vi "minivia.vi"(7 "Minify Locals?":bool, 9 "Remove JavaScriptInvoke":bool=TRUE, 10 "Remove Whitespace":bool, 11 "VIA":string="// Autogenerated Vireo assembly file\n// Generated on 07/31/2021 00:31:29\n//---------------------------------------------------\n//VI Definition: ::Web Server::Interactive::HelloBlink::HelloBlink.gviweb\ndefine (HelloBlink%3A%3AHelloBlink%2Egviweb dv(.VirtualInstrument (\n    Locals: c(   // Data Space\n        e(dv(.String 'HelloBlink::HelloBlink.gviweb')local0)\n        ce(dv(.Boolean true)c1)\n        ce(dv(.UInt32 25)c2)\n        e(.Int32 local3)\n        ce(dv(.Boolean false)c4)\n        ce(dv(.UInt32 1000)c5)\n        ce(dv(.String 'Hello LabWorld %d')c6)\n        e(.String local7)\n        e(.UInt32 local8)\n        e(.UInt32 local9)\n        e(.UInt32 local10)\n        e(.Int32 local11)\n        e(.Boolean local12)\n        e(.Boolean local13)\n        e(.Boolean local14)\n        ce(dv(.Boolean false)c15)\n        ce(dv(.UInt32 500)c16)\n        e(.UInt32 local17)\n        e(.UInt32 local18)\n        ce(dv(.Int32 0)c19)\n        e(.Int32 local20)\n        ce(dv(.Int32 2147483647)c21)\n        ce(dv(.Int32 0)c22)\n        e(.UInt32 local23)\n        ce(dv(.Int32 2147483647)c24)\n    )\n        clump(1\n        Trigger(1)\n        Trigger(2)\n        Wait(1)\n        Wait(2)\n/* Clump Ended. */    )\n    clump(1\n        PicoGLib%3A%3AGPIO%3A%3AInit%2Egvi(c2 local9)\n        PicoGLib%3A%3AGPIO%3A%3ASetOutput%2Egvi(local9 c1 local10)\n        Copy(c1 local13)\n        Copy(c22 local11)\n        Copy(local10 local23)\n    Perch(0)\n        Copy(local13 local12)\n        Not(local12 local14 )\n        Trigger(5)\n        Trigger(6)\n        Wait(5)\n        Wait(6)\n        Copy(local14 local13)\n        BranchIfTrue(1 c15)\n        BranchIfEQ(0 local11 c24)\n        Increment(local11 local11 )\n        Branch(0)\n    Perch(1)\n        // Code End\n/* Clump Ended. */    )\n    clump(1\n        Copy(c19 local3)\n    Perch(0)\n        StringFormatValue(local7 c6 local3 )\n        Trigger(3)\n        Trigger(4)\n        Wait(3)\n        Wait(4)\n        Copy(local3 local20)\n        BranchIfTrue(1 c4)\n        BranchIfEQ(0 local3 c21)\n        Increment(local3 local3 )\n        Branch(0)\n    Perch(1)\n        // Code End\n/* Clump Ended. */    )\n    clump(1\n        PicoGLib%3A%3ACore%3A%3APrintln%2Egvi(local7)\n        // Code End\n/* Clump Ended. */    )\n    clump(1\n        WaitMilliseconds(c5 * )\n        // Code End\n/* Clump Ended. */    )\n    clump(1\n        PicoGLib%3A%3AGPIO%3A%3AWrite%2Egvi(local10 local12 *)\n        // Code End\n/* Clump Ended. */    )\n    clump(1\n        WaitMilliseconds(c16 * )\n        // Code End\n/* Clump Ended. */    )\n)))\n// Autogenerated Vireo assembly file\n// Generated on 07/31/2021 00:29:56\n//---------------------------------------------------\n//VI Definition: ::Web Server::Interactive::PicoGLib::GPIO::Write.gvi\ndefine (PicoGLib%3A%3AGPIO%3A%3AWrite%2Egvi dv(.VirtualInstrument (\n    Params: c(  //param block\n        i(dv(.UInt32 0)dataItem_PinIn)\n        i(dv(.Boolean false)dataItem_Value)\n        o(dv(.UInt32 0)dataItem_PinPinIn)\n    )\n    Locals: c(   // Data Space\n        e(dv(.String 'PicoGLib::GPIO::Write.gvi')local3)\n        e(.Boolean local4)\n        e(.UInt32 local5)\n        e(.UInt32 local6)\n    )\n        clump(1\n        Copy(dataItem_PinIn local5)\n        Copy(local5 dataItem_PinPinIn)\n/* Clump Ended. */    )\n)))\n// Autogenerated Vireo assembly file\n// Generated on 07/31/2021 00:29:56\n//---------------------------------------------------\n//VI Definition: ::Web Server::Interactive::PicoGLib::GPIO::SetOutput.gvi\ndefine (PicoGLib%3A%3AGPIO%3A%3ASetOutput%2Egvi dv(.VirtualInstrument (\n    Params: c(  //param block\n        i(dv(.UInt32 0)dataItem_PinIn)\n        i(dv(.Boolean false)dataItem_Output)\n        o(dv(.UInt32 0)dataItem_PinPinIn)\n    )\n    Locals: c(   // Data Space\n        e(dv(.String 'PicoGLib::GPIO::SetOutput.gvi')local3)\n        e(.Boolean local4)\n        e(.UInt32 local5)\n        e(.UInt32 local6)\n    )\n        clump(1\n        Copy(dataItem_PinIn local5)\n        Copy(local5 dataItem_PinPinIn)\n/* Clump Ended. */    )\n)))\n// Autogenerated Vireo assembly file\n// Generated on 07/31/2021 00:29:56\n//---------------------------------------------------\n//VI Definition: ::Web Server::Interactive::PicoGLib::GPIO::Init.gvi\ndefine (PicoGLib%3A%3AGPIO%3A%3AInit%2Egvi dv(.VirtualInstrument (\n    Params: c(  //param block\n        i(dv(.UInt32 0)dataItem_PinIn)\n        o(dv(.UInt32 0)dataItem_PinPinIn)\n    )\n    Locals: c(   // Data Space\n        e(dv(.String 'PicoGLib::GPIO::Init.gvi')local2)\n        e(.UInt32 local3)\n        e(.UInt32 local4)\n    )\n        clump(1\n        Copy(dataItem_PinIn local3)\n        Copy(local3 dataItem_PinPinIn)\n/* Clump Ended. */    )\n)))\n// Autogenerated Vireo assembly file\n// Generated on 07/31/2021 00:31:10\n//---------------------------------------------------\n//VI Definition: ::Web Server::Interactive::PicoGLib::Core::Println.gvi\ndefine (PicoGLib%3A%3ACore%3A%3APrintln%2Egvi dv(.VirtualInstrument (\n    Params: c(  //param block\n        i(dv(.String '')dataItem_String)\n    )\n    Locals: c(   // Data Space\n        e(dv(.String 'PicoGLib::Core::Println.gvi')local1)\n        e(.String local2)\n    )\n        clump(1\n/* Clump Ended. */    )\n)))\nenqueue (HelloBlink%3A%3AHelloBlink%2Egviweb)\n//Finished!! :D\n") -> (3 "Minified":string)   [LabVIEW 2020]
uses:
  <vilib>/regexp/Match Regular Expression.xnode
panel:
  out "% saved":dbl
  out "length":i32
  in  "Remove Enqueue?":bool
  in  "Rename Top-Level (Blank = as-is)":string="main"
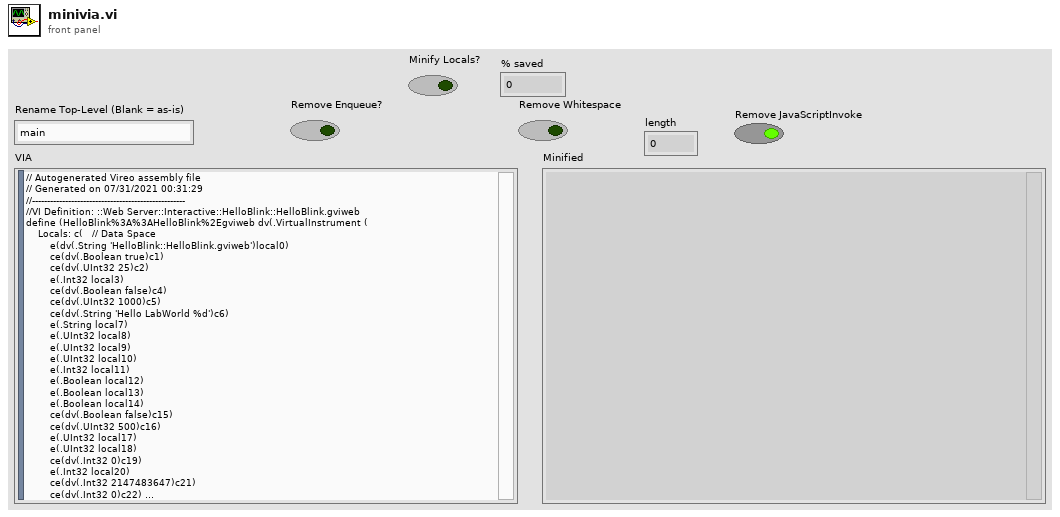
[diagram p1: front panel]
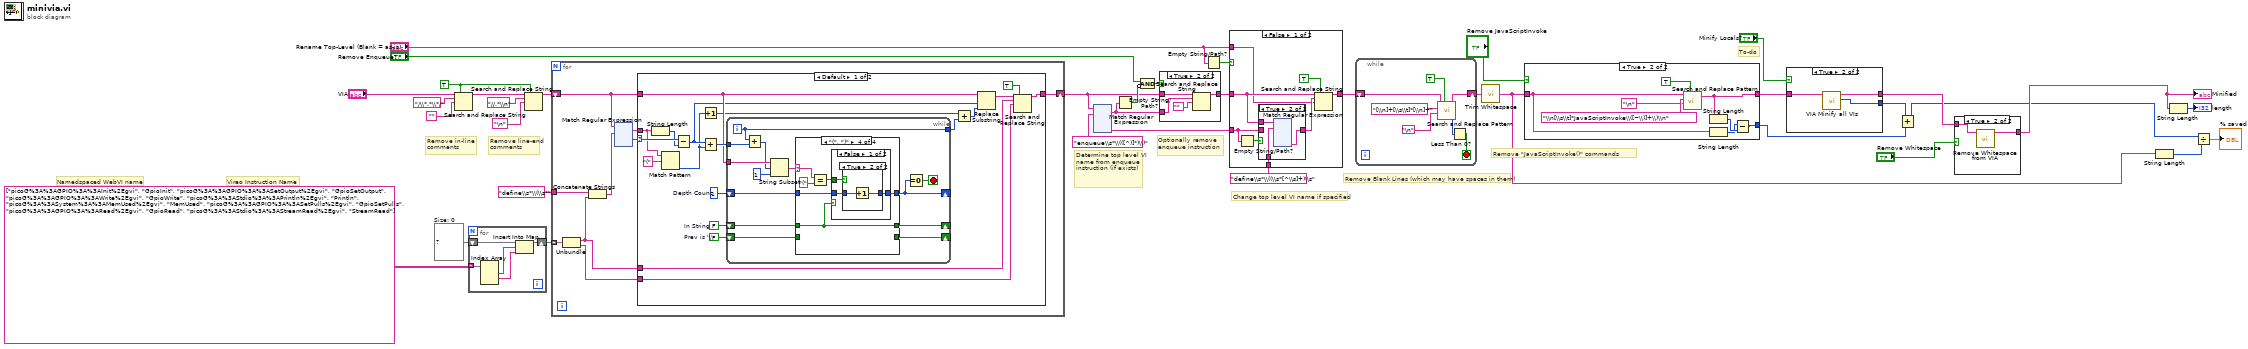
[diagram p0: block diagram]
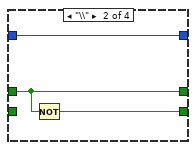
[diagram p6: hidden frame]
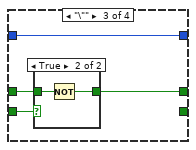
[diagram p7: hidden frame]
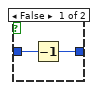
[diagram p9: hidden frame]
diagram:
  w17 = map{string, string} {}  # Size: 0
  w34 = TRUE ("replace all? (F)")
  # "Remove \"JavaScriptInvoke()\" commands"
  # "Remove Blank Lines (which may have spaces in them)"
  # "Vireo Instruction Name"
  # "Namedspaced WebVI name"
  # "To-do"
  # "Change top level VI name if specified"
  # "Optionally remove enqueue instruction"
  # "Determine top level VI name from enqueue instruction (if exists)"
  # "Remove line-end comments"
  # "Remove in-line comments"
  n1 = Search and Replace String(replace all?=w34, input string="VIA", search string="/\\*.*\\*/", replace string="") -> (result string=w36:string)  [unwired: 4 in, 3 out]
  n2 = for {
    tunnel: string[][] [["picoG%3A%3AGPIO%3A%3AInit%2Egvi", "GpioInit"], ["picoG%3A%3AGPIO%3A%3ASetOutput%2Egvi", "GpioSetOutput"], ["picoG%3A%3AGPIO%3A%3AWrite%2Egvi", "GpioWrite"], ["picoG%3A%3AStdio%3A%3APrintln%2Egvi", "Println"], ["picoG%3A%3ASystem%3A%3AMemUsed%2Egvi", "MemUsed"], ["picoG%3A%3AGPIO%3A%3ASetPulls%2Egvi", "GpioSetPulls"], ["picoG%3A%3AGPIO%3A%3ARead%2Egvi", "GpioRead"], ["picoG%3A%3AStdio%3A%3AStreamRead%2Egvi", "StreamRead"]] -> [w42] mode=indexing
    shift-right: [w40] -> w20
    shift-left: w17 -> [w43]
    n3 = Index Array(array=w42) -> (element #1=w41:string, element #2=w39:string)  [unwired: 3 in, 1 out]
    n4 = Insert Into Map(map in=w43, key=w41, value=w39) -> (map out=w40:map{string, string})  [unwired: 2 out]
  }
  n5 = Search and Replace String(replace all?=w34, input string=w36, search string="//.*\\n", replace string="\n") -> (result string=w21:string)  [unwired: 4 in, 3 out]
  n6 = for {
    shift-right: [w47] -> w18
    shift-left: w21 -> [w48]
    tunnel: w20 -> [w52] mode=indexing
    tunnel: "define\\s*\\(\\s*" -> [w51]
    n7 = Unbundle(w52) -> (w44:string, w45:string)
    n8 = Concatenate Strings(w51, w44) -> (w50:string)
    n9 = xnode "Match Regular Expression"("input string"=w48, "regular expression"=w50) -> ("whole match"=w46:string, "offset past match"=w49:i32)  [unwired: 4 in, 3 out]
    n10 = case shown="Default" w49 {
      selector: w49 -> [w71 _]
      tunnel: w48 -> [w64 w111]
      tunnel: [w54 w111] -> w47
      tunnel: w46 -> [w69 _]
      tunnel: w45 -> [w58 _]
      tunnel: w44 -> [w56 _]
      frame Default {
        w53 = FALSE  # Prev is '\'
        w65 = FALSE  # In String
        w67 = 1  # Depth Count
        n11 = String Length(string=w69) -> (length=w70:i32)
        n12 = Match Pattern(string=w69, regular expression="(") -> (offset past match=w61:i32)  [unwired: 1 in, 3 out]
        n13 = Subtract(x=w71, y=w70) -> (x-y=w63:i32)
        n14 = Increment(x=w61) -> (x+1=w59:i32)
        n15 = Add(x=w63, y=w61) -> (x+y=w66:i32)
        n16 = while {
          shift-right: [w76] -> _
          shift-left: w67 -> [w80]
          tunnel: w66 -> [w84]
          tunnel: w64 -> [w83]
          shift-right: [w73] -> _
          shift-left: w65 -> [w78]
          shift-right: [w74] -> _
          shift-left: w53 -> [w77]
          tunnel: [w72] -> w62
          i -> [w72]
          stop <- w75 stop-if-true
          n17 = Add(x=w72, y=w84) -> (x+y=w82:i32)
          n18 = String Subset(string=w83, offset (0)=w82, length (rest)=1 ("length (rest)")) -> (substring=w79:string)
          n19 = case shown="\"(\", \")\"" w79 {
            selector: w79 -> [_ _ _ w100]
            tunnel: w80 -> [w86 w88 w90 w102]
            tunnel: [w86 w88 w90 w101] -> w76
            tunnel: w78 -> [w85 w87 w92 w98]
            tunnel: w77 -> [_ _ w93 _]
            tunnel: [_ w89 _ _] -> w74
            tunnel: [w85 w87 w91 w98] -> w73
            frame Default {
            }
            frame "\\" {
              n20 = Not(x=w87) -> (.not. x?=w89:bool)
            }
            frame "\"" {
              n21 = case shown="True" w93 {
                tunnel: w92 -> [w94 w96]
                tunnel: [w94 w95] -> w91
                frame False {
                }
                frame True {
                  n22 = Not(x=w96) -> (.not. x?=w95:bool)
                }
              }
            }
            frame "(", ")" {
              n23 = Equal?(x=w100, y="(") -> (x = y?=w97:bool)
              n24 = case shown="False" w98 {
                tunnel: w102 -> [w105 w110]
                tunnel: [w104 w110] -> w101
                tunnel: w97 -> [w103 _]
                frame False {
                  n25 = case shown="True" w103 {
                    tunnel: w105 -> [w107 w109]
                    tunnel: [w106 w108] -> w104
                    frame False {
                      n26 = Decrement(x=w107) -> (x-1=w106:i32)
                    }
                    frame True {
                      n27 = Increment(x=w109) -> (x+1=w108:i32)
                    }
                  }
                }
                frame True {
                }
              }
            }
          }
          n28 = Equal To 0?(x=w76) -> (x = 0?=w75:bool)
        }
        n29 = Add(x=w59, y=w62) -> (x+y=w60:i32)
        n30 = Replace Substring(2:w60, 3:w63, 5:w64) -> (1:w57:string)  [unwired: 1 in, 1 out]
        n31 = Search and Replace String(replace all?=TRUE ("replace all? (F)"), input string=w57, search string=w56, replace string=w58) -> (result string=w54:string)  [unwired: 4 in, 3 out]
      }
      frame -1 {
        # "Built-in not used"
      }
    }
  }
  n32 = xnode "Match Regular Expression"("input string"=w18, "regular expression"="enqueue\\s*\\(([^)]*)\\)") -> ("whole match"=w30:string, "submatch 1"=w27:string)  [unwired: 4 in, 4 out]
  n33 = Empty String/Path?(string/path=w30) -> (empty?=w29:bool)
  n34 = Compound Arithmetic op=AND("Remove Enqueue?", invert w29) -> (w28:bool)
  n35 = case shown="True" w28 {
    tunnel: w18 -> [w226 w230]
    tunnel: w30 -> [_ w228]
    tunnel: [w226 w229] -> w26
    frame False {
    }
    frame True {
      n36 = Search and Replace String(input string=w230, search string=w228, replace string="") -> (result string=w229:string)  [unwired: 5 in, 3 out]
    }
  }
  n37 = Empty String/Path?(string/path="Rename Top-Level (Blank = as-is)") -> (empty?=w25:bool)
  n38 = case shown="False" w25 {
    tunnel: w27 -> [w236 _]
    tunnel: w26 -> [w235 w359]
    tunnel: [w234 w359] -> w15
    tunnel: "define\\s*\\((\\s*[^\\s]+)\\s" ("regular expression") -> [w237 _]
    tunnel: "Rename Top-Level (Blank = as-is)" -> [w231 _]
    frame False {
      n39 = Empty String/Path?(string/path=w236) -> (empty?=w238:bool)
      n40 = case shown="True" w238 {
        tunnel: w235 -> [_ w242]
        tunnel: w237 -> [_ w241]
        tunnel: w236 -> [w239 _]
        tunnel: [w239 w240] -> w232
        frame False {
        }
        frame True {
          n41 = xnode "Match Regular Expression"("input string"=w242, "regular expression"=w241) -> ("submatch 1"=w240:string)  [unwired: 4 in, 5 out]
        }
      }
      n42 = Search and Replace String(replace all?=TRUE ("replace all? (F)"), input string=w235, search string=w232, replace string=w231) -> (result string=w234:string)  [unwired: 4 in, 3 out]
    }
    frame True {
    }
  }
  n43 = while {
    shift-right: [w363] -> w6
    shift-left: w15 -> [w364]
    stop <- w360 stop-if-true
    n44 = call <vilib>:"Search and Replace Pattern.vi"("string"=w364, "regular expression (\"\")"="[\\n]+[\\s\\t]*[\\n]+" ("regular expression (\"\")"), "replace string (\"\")"="\n", "replace all? (F)"=TRUE) -> ("result string"=w363:string, "offset past match"=w361:i32)  [unwired: 1 in]
    n45 = Less Than 0?(x=w361) -> (x < 0?=w360:bool)
  }
  n46 = call <vilib>:"Trim Whitespace.vi"("string"=w6) -> ("trimmed string"=w4:string)  [unwired: 1 in]
  n47 = case shown="True" "Remove JavaScriptInvoke" {
    tunnel: w4 -> [w367 w371]
    tunnel: [w367 w372] -> w5
    tunnel: [_ w368] -> w3
    frame False {
    }
    frame True {
      n48 = call <vilib>:"Search and Replace Pattern.vi"("string"=w371, "regular expression (\"\")"="\\n[\\s\\t]*JavaScriptInvoke\\([~\\)]+\\)\\n" ("regular expression (\"\")"), "replace string (\"\")"="\n" ("replace string (\"\")"), "replace all? (F)"=TRUE) -> ("result string"=w372:string)  [unwired: 1 in, 1 out]
      n49 = String Length(string=w372) -> (length=w370:i32)
      n50 = String Length(string=w371) -> (length=w369:i32)
      n51 = Subtract(x=w369, y=w370) -> (x-y=w368:i32)
    }
  }
  n52 = case shown="True" "Minify Locals?" {
    tunnel: w5 -> [w376 w379]
    tunnel: [w376 w378] -> w8
    tunnel: [_ w377] -> w2
    frame False {
    }
    frame True {
      n53 = call "VIA Minify all VIs.vi"("VIA in"=w379) -> ("Bytes Removed"=w377:i32, "VIA out"=w378:string)  [unwired: 9 in]
    }
  }
  n54 = Add(x=w2, y=w3) -> (x+y=w1:i32)
  n55 = case shown="True" "Remove Whitespace" {
    tunnel: [w380 w382] -> w7
    tunnel: w8 -> [w380 w381]
    frame False {
    }
    frame True {
      n56 = call "Remove Whitespace from VIA.vi"("Pretty Printed VIA"=w381) -> ("Ugly Printed VIA"=w382:string)  [unwired: 10 in]
    }
  }
  "Minified" <- w7
  n57 = String Length(string=w4) -> (length=w9:i32)
  n58 = String Length(string=w7) -> (length=→"length":i32)
  n59 = Divide(x=w1, y=w9) -> (x/y=→"% saved":dbl)
